vi "Get External Trigger Mode.vi"(8 "error in (no error)":errorcluster, 11 "hdl":i32) -> (0 "error out":errorcluster, 2 "External Trigger Mode":T1, 3 "hdl out":i32)   [LabVIEW 2013, in "Thorlabs_SC10.lvlib"]
uses:
  <instrlib>/Thorlabs_SC10/Thorlabs_SC10.lvlib
  <instrlib>/Thorlabs_SC10/Public/Configure/External Trigger Mode.ctl
  <instrlib>/Thorlabs_SC10/Data/SC10CommandLib_x64.dll
  <instrlib>/Thorlabs_SC10/Data/SC10CommandLib_win32.dll
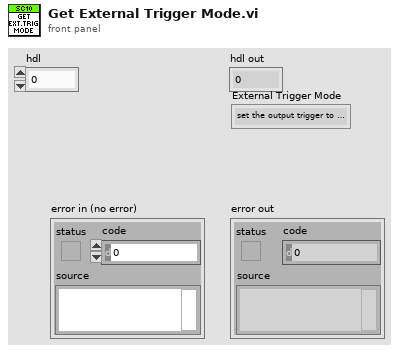
[diagram p1: front panel]
types:
  T1 = typedef "Thorlabs_SC10.lvlib/External Trigger Mode.ctl" = enum16{"set the output trigger to follow the shutter output when the SH05 is connected", "force the trigger output to follow the controller output when an SH05 is equipped"}
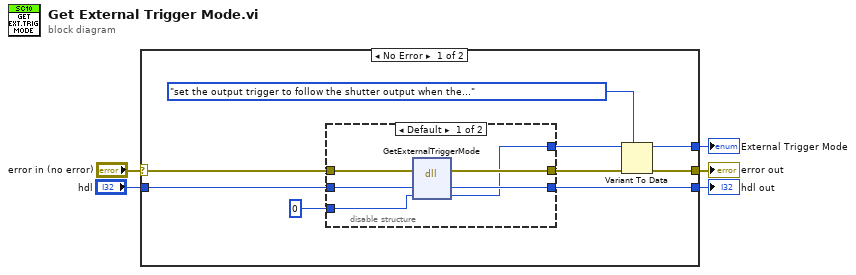
[diagram p0: block diagram]
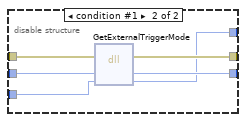
[diagram p2: hidden frame]
diagram:
  n1 = case shown="No Error" "error in (no error)" {
    selector: "error in (no error)" -> [w14 w27]
    tunnel: [w10 w27] -> w5
    tunnel: "hdl" -> [w12 _]
    tunnel: [w11 _] -> w2
    tunnel: [w7 _] -> w1
    frame No Error {
      n2 = disable-structure shown="Default" {
        disable-tunnel: w14 -> [w20 w26]
        disable-tunnel: [w19 w25] -> w13
        disable-tunnel: w12 -> [w18 w24]
        disable-tunnel: [w17 w23] -> w11
        disable-tunnel: [w16 w21] -> w9
        disable-tunnel: 0 ("value") -> [w15 w22]
        frame condition #0 (active) {
          n3 = dll-call lib="C:/Program Files (x86)/National Instruments/LabVIEW 2013/instr.lib/Thorlabs_SC10/Data/SC10CommandLib_win32.dll" fn="GetExternalTriggerMode"(error in=w20, "hdl"=w18, "value"=w15) -> (error out=w19:errorcluster, "hdl"=w17:i32, "value"=w16:i32)  [unwired: 3 in, 1 out]
        }
        frame condition #1 {
          n4 = dll-call lib="C:/Program Files/National Instruments/LabVIEW 2013/instr.lib/Thorlabs_SC10/Data/SC10CommandLib_x64.dll" fn="GetExternalTriggerMode"(error in=w26, "hdl"=w24, "value"=w22) -> (error out=w25:errorcluster, "hdl"=w23:i32, "value"=w21:i32)  [unwired: 3 in, 1 out]
        }
      }
      n5 = Variant To Data(error in=w13, type=External_Trigger_Mode."set the output trigger to follow the shutter output when the SH05 is connected" ("External Trigger Mode"), Variant=w9) -> (data=w7:T1, error out=w10:errorcluster)
    }
    frame Error {
    }
  }
  "error out" <- w5
  "hdl out" <- w2
  "External Trigger Mode" <- w1
